vi "Add_Next_Calib_Details.vi"(1 "% Change":dbl format="%.2f", 3 "Hours between calibrations":dbl format="%.2f", 4 "Instrument type":T1=enum."Cross wire velocity", 5 "Calib file Orig":path=path "/Hong(6%)/calib/XW Ch 1 7_10_02_5", 6 "Calib file New":path=path "/Hong(6%)/calib/XW Ch 1 7_10_02_6") -> (0 "Results Files Updated":bool)   [LabVIEW 2010]
uses:
  Controls/Cal_Inst_type.ctl
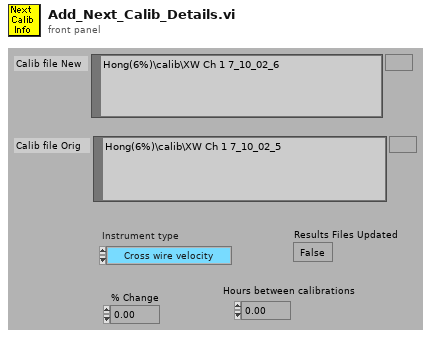
[diagram p1: front panel]
types:
  T1 = typedef "Cal_Inst_type.ctl" = enum16{"Propeller anemometer", "Pressure Transducer", "Hot wire", "Cross wire velocity", "Cross wire angle", "Generic Linear", "Generic Polynomial", "Generic BackPoly", "Fast FID", "Thermocouple", "Cold wire", "Pulsed Wire"}
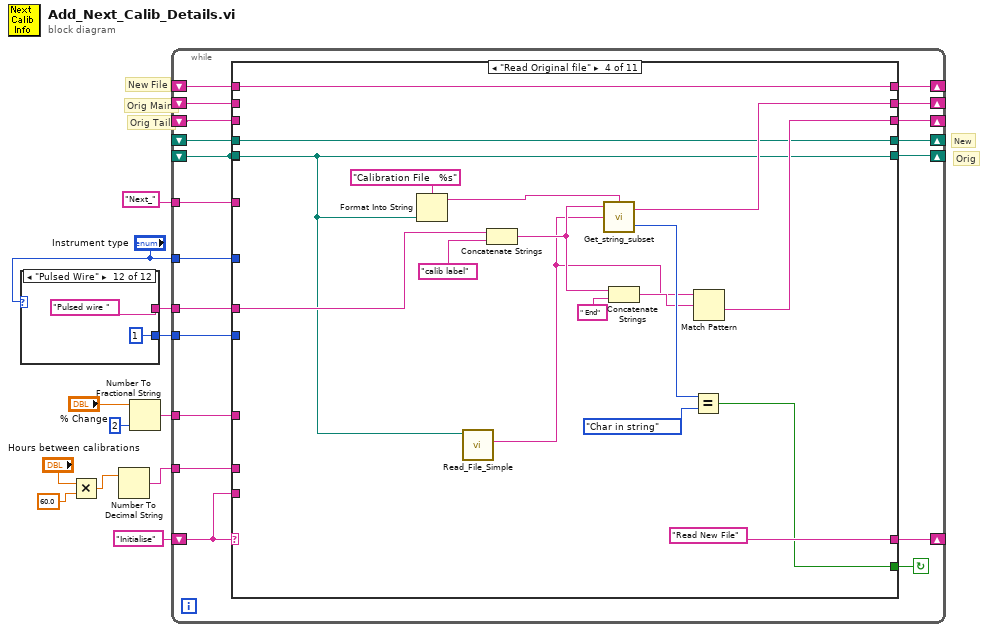
[diagram p0: block diagram]
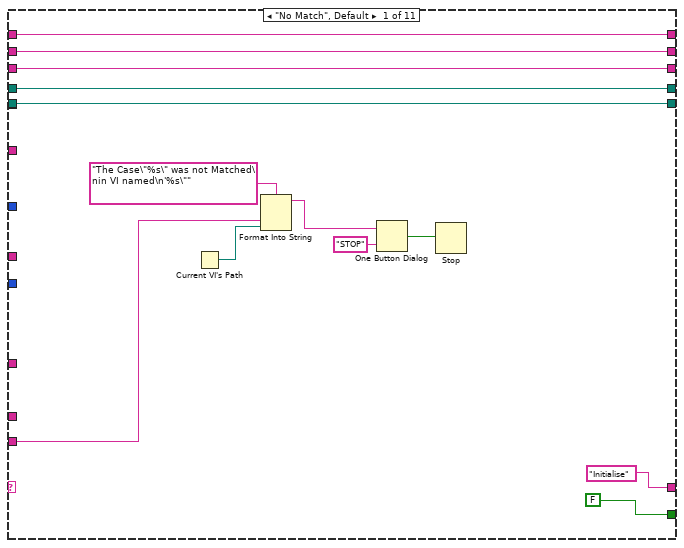
[diagram p2: hidden frame]
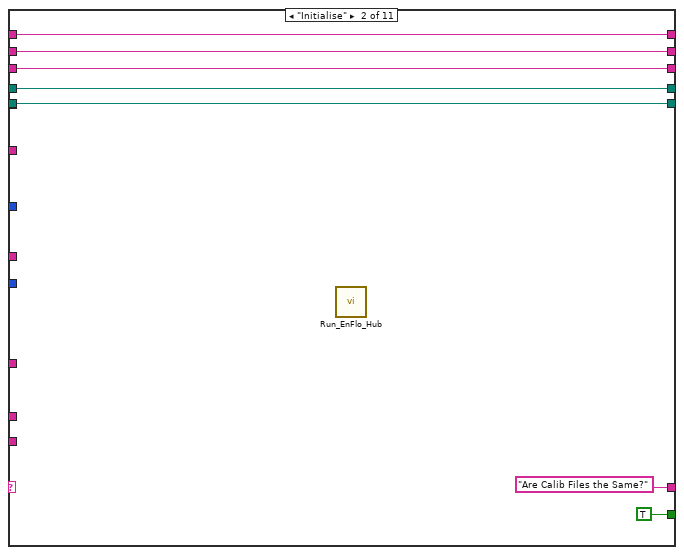
[diagram p3: hidden frame]
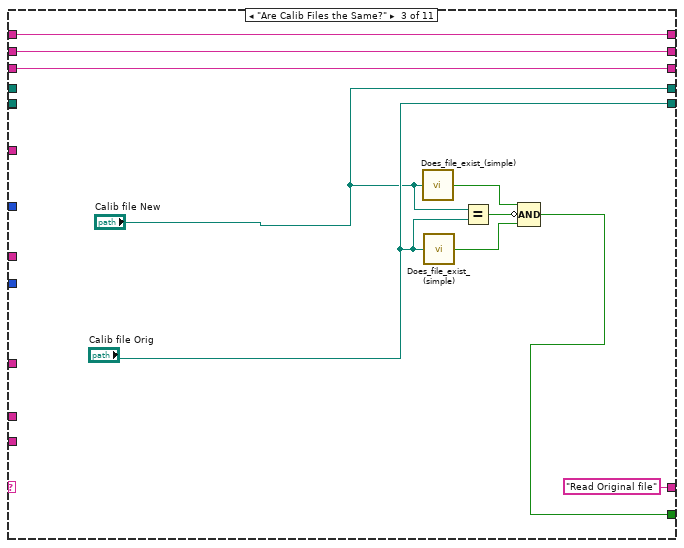
[diagram p4: hidden frame]
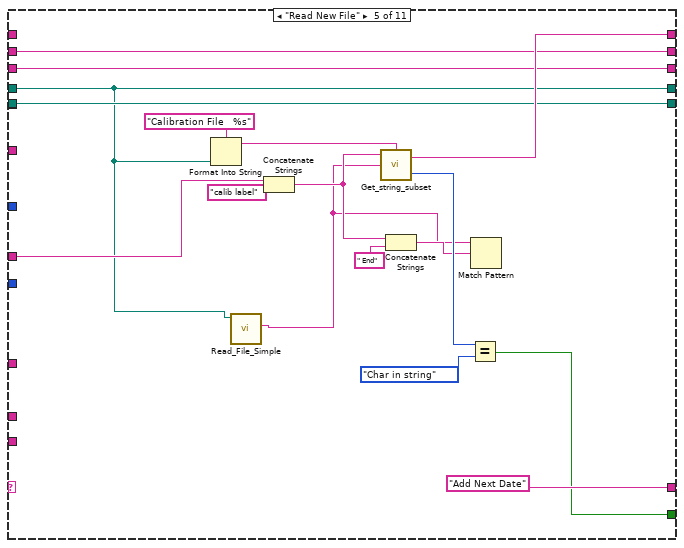
[diagram p5: hidden frame]
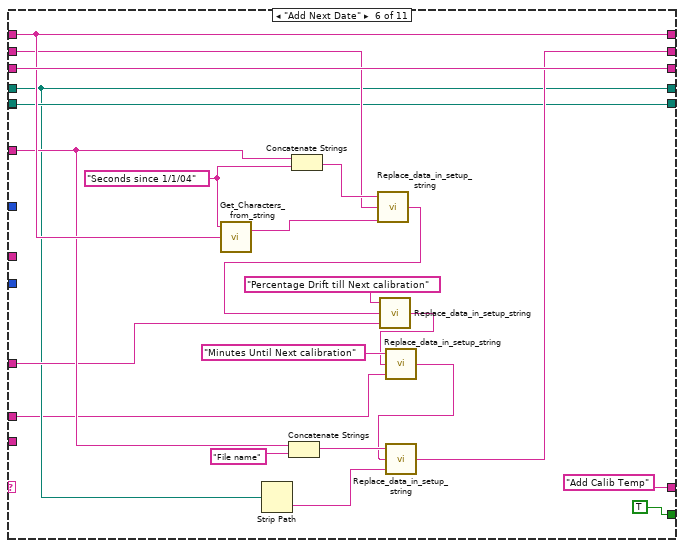
[diagram p6: hidden frame]
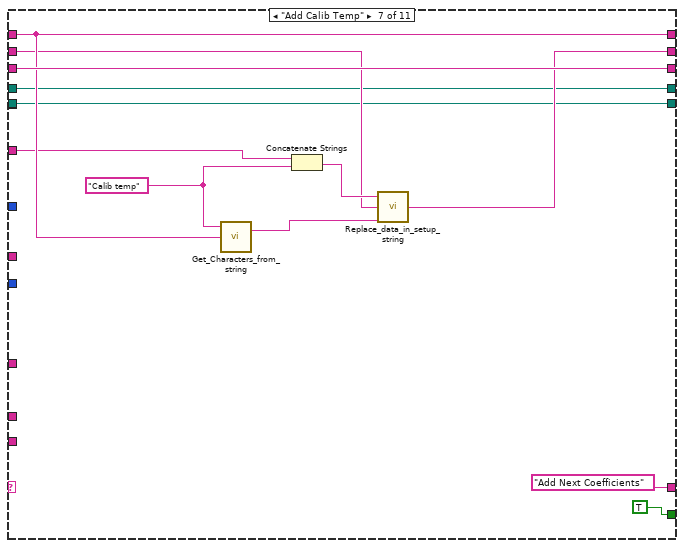
[diagram p7: hidden frame]
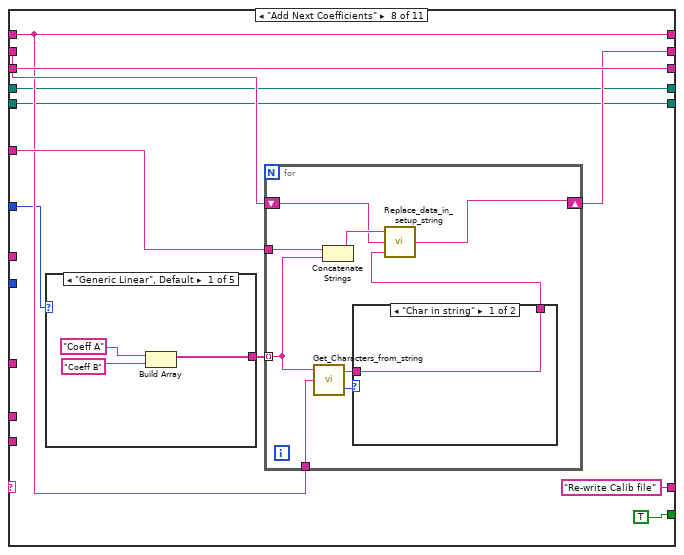
[diagram p8: hidden frame]
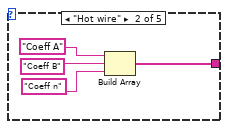
[diagram p9: hidden frame]
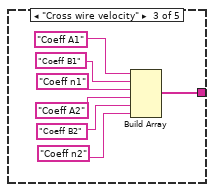
[diagram p10: hidden frame]
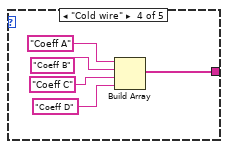
[diagram p11: hidden frame]
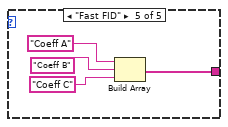
[diagram p12: hidden frame]
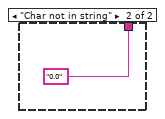
[diagram p13: hidden frame]
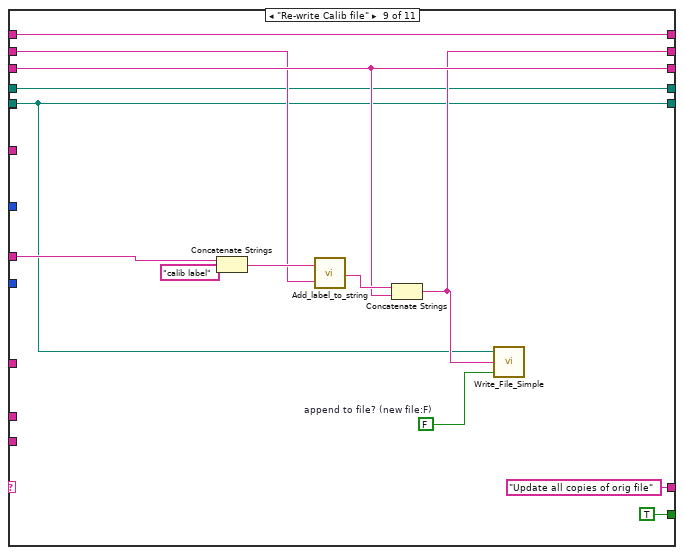
[diagram p14: hidden frame]
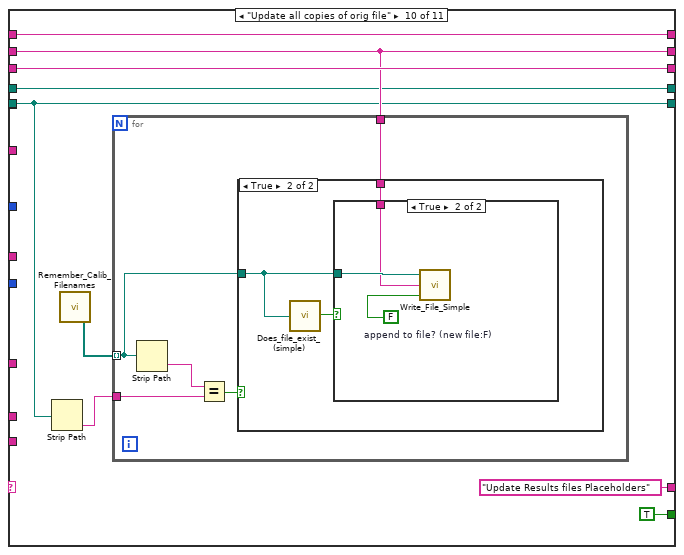
[diagram p15: hidden frame]
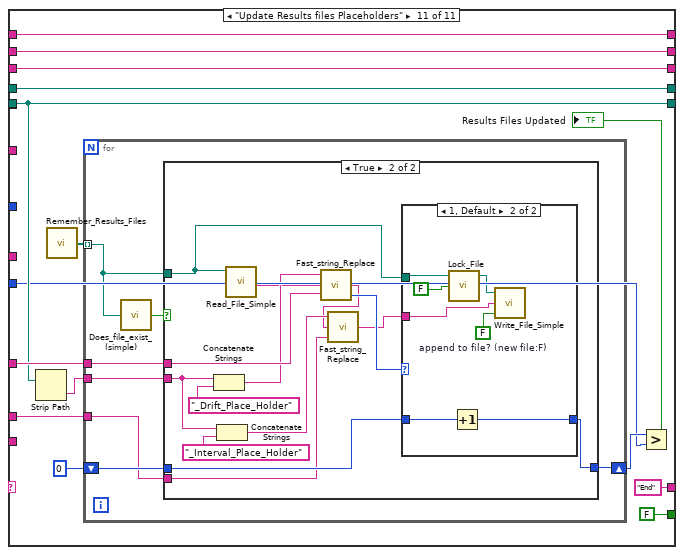
[diagram p18: hidden frame]
diagram:
  # "Orig"
  # "New"
  # "Orig Tail"
  # "New File"
  # "Orig Main"
  n1 = case shown="\"Pulsed Wire\"" "Instrument type" {
    tunnel: ["Prop " "Mano " "HW " "Cross wire velocity " "Cross wire angle " "Generic Inst " "Generic Polynomial " "Generic BackPoly " "Fast FID " "Thermocouple " "Cold wire " "Pulsed wire "] -> w10
    tunnel: [1 ("y") 1 ("y") 1 ("y") 1 ("y") 1 ("y") 1 ("y") 1 ("y") 1 ("y") 3 ("y") 1 ("y") 1 ("y") 1 ("y")] -> w1
    frame "Propeller anemometer" {
    }
    frame "Pressure Transducer" {
    }
    frame "Hot wire" {
    }
    frame "Cross wire velocity" {
    }
    frame "Cross wire angle" {
    }
    frame "Generic Linear" {
    }
    frame "Generic Polynomial" {
    }
    frame "Generic BackPoly" {
    }
    frame "Fast FID" {
    }
    frame "Thermocouple" {
    }
    frame "Cold wire" {
    }
    frame "Pulsed Wire" {
    }
  }
  n2 = Multiply(x="Hours between calibrations", y=60.0) -> (x*y=w3:dbl)
  n3 = Number To Decimal String(number=w3) -> (decimal integer string=w5:string)  [unwired: 1 out]
  n4 = Number To Fractional String(number="% Change", precision (6)=i16 2) -> (F-format string=w6:string)  [unwired: 2 out]
  n5 = while {
    shift-left: _ -> [w39]
    shift-right: [w41] -> _
    shift-left: _ -> [w42]
    shift-right: [w40] -> _
    tunnel: w6 -> [w43]
    tunnel: "Next_" -> [w44]
    tunnel: w10 -> [w45]
    shift-left: _ -> [w46]
    shift-right: [w47] -> _
    shift-left: _ -> [w48]
    shift-right: [w50] -> _
    tunnel: "Instrument type" -> [w52]
    shift-left: _ -> [w49]
    shift-right: [w51] -> _
    shift-left: "Initialise" -> [w53]
    shift-right: [w54] -> _
    tunnel: w5 -> [w38]
    tunnel: w1 -> [w37]
    stop <- w55 continue-if-true
    n6 = case shown="\"Read Original file\"" w53 {
      tunnel: [FALSE TRUE w78 w91 w108 TRUE TRUE TRUE TRUE TRUE FALSE] -> w55
      tunnel: ["Initialise" "Are Calib Files the Same?" "Read Original file" "Read New File" "Add Next Date" "Add Calib Temp" "Add Next Coefficients" "Re-write Calib file" "Update all copies of orig file" "Update Results files Placeholders" "End"] -> w54
      tunnel: w53 -> [w63 _ _ _ _ _ _ _ _ _ _]
      tunnel: w52 -> [_ _ _ _ _ _ _ w157 _ _ _]
      tunnel: [w60 w75 w85 w95 w117 w135 w147 w158 w209 w218 w244] -> w51
      tunnel: [w59 w73 w83 w93 w110 w136 w148 w164 w204 w217 w243] -> w50
      tunnel: w49 -> [w60 w75 w85 w95 _ w135 w147 w158 w209 w218 w244]
      tunnel: w48 -> [w59 w73 w83 _ w110 w136 w148 w164 w204 w217 w243]
      tunnel: [w58 w74 w84 w94 w111 w131 w144 w159 w201 w214 w241] -> w47
      tunnel: w46 -> [w58 w74 w84 _ w111 w134 w146 w160 w202 w214 w241]
      tunnel: w45 -> [_ _ _ w99 w114 _ _ _ w207 _ _]
      tunnel: w44 -> [_ _ _ _ _ w129 w145 w161 _ _ _]
      tunnel: w43 -> [_ _ _ _ _ w126 _ _ _ _ w239]
      tunnel: [w57 w70 "Calib file New" w90 w104 w124 w143 w155 w200 w213 w238] -> w40
      tunnel: [w56 w69 "Calib file Orig" w86 w107 w125 w142 w154 w199 w212 w237] -> w41
      tunnel: w39 -> [w56 w69 _ w86 w107 w125 w142 w154 w199 w212 _]
      tunnel: w42 -> [w57 w70 _ w90 w104 w124 w143 w155 w200 w213 w238]
      tunnel: w39 -> [_ _ _ _ _ _ _ _ _ _ w237]
      tunnel: w38 -> [_ _ _ _ _ w120 _ _ _ _ w235]
      tunnel: w37 -> [_ _ _ _ _ _ _ _ _ _ w232]
      frame "No Match", Default {
        n7 = Current VI's Path() -> (path=w62:path)
        n8 = Format Into String(format string="The Case\"%s\" was not Matched\nin VI named\n'%s\"" ("Format String"), w63, w62) -> (resulting string=w66:string)  [unwired: 2 in, 1 out]
        n9 = One Button Dialog(message=w66, button name ("OK")="STOP") -> (true=w64:bool)
        n10 = Stop(stop? (T)=w64) -> ()
      }
      frame "Initialise" {
        n11 = call "Run_EnFlo_Hub.vi"() -> ()  [unwired: 8 out]
      }
      frame "Are Calib Files the Same?" {
        n12 = call "Does_file_exist_(simple).vi"("Pathname"="Calib file New") -> ("exists?"=w80:bool)
        n13 = call "Does_file_exist_(simple).vi"("Pathname"="Calib file Orig") -> ("exists?"=w79:bool)
        n14 = Equal?(x="Calib file New", y="Calib file Orig") -> (x = y?=w81:bool)
        n15 = Compound Arithmetic op=AND(w80, invert w81, w79) -> (w78:bool)
      }
      frame "Read Original file" {
        n16 = Format Into String(format string="Calibration File   %s", w86) -> (resulting string=w87:string)  [unwired: 2 in, 1 out]
        n17 = call "Read_File_Simple.vi"("Filename"=w86) -> ("string"=w89:string)  [unwired: 2 in, 7 out]
        n18 = Concatenate Strings(w99, "calib label") -> (w96:string)
        n19 = call "Get_string_subset.vi"("String Name"=w87, "String to split"=w89, "File Label"=w96) -> ("Status"=w100:enum16{"Char in string", "Char not in string"}, "Output string"=w94:string)  [unwired: 1 in]
        n20 = Concatenate Strings(w96, " End") -> (w97:string)
        n21 = Equal?(x=w100, y=enum16{"Char in string", "Char not in string"}."Char in string" ("Status")) -> (x = y?=w91:bool)
        n22 = Match Pattern(string=w89, regular expression=w97) -> (after substring=w93:string)  [unwired: 4 out]
      }
      frame "Read New File" {
        n23 = Format Into String(format string="Calibration File   %s", w104) -> (resulting string=w103:string)  [unwired: 2 in, 1 out]
        n24 = call "Read_File_Simple.vi"("Filename"=w104) -> ("string"=w106:string)  [unwired: 2 in, 7 out]
        n25 = Concatenate Strings(w114, "calib label") -> (w109:string)
        n26 = call "Get_string_subset.vi"("String Name"=w103, "String to split"=w106, "File Label"=w109) -> ("Status"=w116:enum16{"Char in string", "Char not in string"}, "Output string"=w117:string)  [unwired: 1 in]
        n27 = Concatenate Strings(w109, " End") -> (w112:string)
        n28 = Equal?(x=w116, y=enum16{"Char in string", "Char not in string"}."Char in string" ("Status")) -> (x = y?=w108:bool)
        n29 = Match Pattern(string=w106, regular expression=w112) -> ()  [unwired: 5 out]
      }
      frame "Add Next Date" {
        w139 = "Seconds since 1/1/04"
        n30 = call "Get_Characters_from_string.vi"("Input string"=w135, "Variable name"=w139) -> ("Value"=w137:string)  [unwired: 1 in, 1 out]
        n31 = Strip Path(path=w124) -> (name=w127:string)  [unwired: 1 out]
        n32 = Concatenate Strings(w129, "File name" ("Variable name")) -> (w128:string)
        n33 = Concatenate Strings(w129, w139) -> (w138:string)
        n34 = call "Replace_data_in_setup_string.vi"("New data string"=w137, "Input string"=w134, "Variable name"=w138) -> ("Appended string"=w132:string)
        n35 = call "Replace_data_in_setup_string.vi"("New data string"=w126, "Input string"=w132, "Variable name"="Percentage Drift till Next calibration") -> ("Appended string"=w122:string)
        n36 = call "Replace_data_in_setup_string.vi"("New data string"=w120, "Input string"=w122, "Variable name"="Minutes Until Next calibration") -> ("Appended string"=w121:string)
        n37 = call "Replace_data_in_setup_string.vi"("New data string"=w127, "Input string"=w121, "Variable name"=w128) -> ("Appended string"=w131:string)
      }
      frame "Add Calib Temp" {
        w151 = "Calib temp"
        n38 = call "Get_Characters_from_string.vi"("Input string"=w147, "Variable name"=w151) -> ("Value"=w149:string)  [unwired: 1 in, 1 out]
        n39 = Concatenate Strings(w145, w151) -> (w150:string)
        n40 = call "Replace_data_in_setup_string.vi"("New data string"=w149, "Input string"=w146, "Variable name"=w150) -> ("Appended string"=w144:string)
      }
      frame "Add Next Coefficients" {
        n41 = case shown="\"Generic Linear\", Default" w157 {
          tunnel: [w165 w168 w172 w179 w184] -> w156
          frame "Generic Linear", Default {
            n42 = Build Array("Coeff A", "Coeff B") -> (w165:string[])
          }
          frame "Hot wire" {
            n43 = Build Array("Coeff A", "Coeff B", "Coeff n") -> (w168:string[])
          }
          frame "Cross wire velocity" {
            n44 = Build Array("Coeff A1", "Coeff B1", "Coeff n1", "Coeff A2", "Coeff B2", "Coeff n2") -> (w172:string[])
          }
          frame "Cold wire" {
            n45 = Build Array("Coeff A", "Coeff B", "Coeff C", "Coeff D") -> (w179:string[])
          }
          frame "Fast FID" {
            n46 = Build Array("Coeff A", "Coeff B", "Coeff C") -> (w184:string[])
          }
        }
        n47 = for {
          tunnel: w156 -> [w195] mode=indexing
          tunnel: w161 -> [w196]
          shift-right: [w192] -> w159
          shift-left: w160 -> [w193]
          tunnel: w158 -> [w188]
          n48 = call "Get_Characters_from_string.vi"("Input string"=w188, "Variable name"=w195) -> ("Status"=w191:enum16{"Char in string", "Char not in string"}, "Value"=w190:string)  [unwired: 1 in]
          n49 = Concatenate Strings(w196, w195) -> (w194:string)
          n50 = case shown="\"Char in string\"" w191 {
            tunnel: w190 -> [w197 _]
            tunnel: [w197 "0.0"] -> w189
            frame "Char in string" {
            }
            frame "Char not in string" {
            }
          }
          n51 = call "Replace_data_in_setup_string.vi"("New data string"=w189, "Input string"=w193, "Variable name"=w194) -> ("Appended string"=w192:string)
        }
      }
      frame "Re-write Calib file" {
        w203 = FALSE  # append to file? (new file:F)
        n52 = Concatenate Strings(w207, "calib label") -> (w206:string)
        n53 = call "Add_label_to_string.vi"("String to write"=w202, "File Label"=w206) -> ("Output string"=w205:string)
        n54 = Concatenate Strings(w205, w204) -> (w201:string)
        n55 = call "Write_File_Simple.vi"("append to file? (new file:F)"=w203, "character string"=w201, "file path"=w199) -> ()  [unwired: 2 out]
      }
      frame "Update all copies of orig file" {
        n56 = Strip Path(path=w212) -> (name=w215:string)  [unwired: 1 out]
        n57 = call "Remember_Calib_Filenames.vi"() -> ("List of Filenames"=w216:path[])  [unwired: 1 in]
        n58 = for {
          tunnel: w216 -> [w222] mode=indexing
          tunnel: w215 -> [w224]
          tunnel: w214 -> [w221]
          n59 = Strip Path(path=w222) -> (name=w225:string)  [unwired: 1 out]
          n60 = Equal?(x=w225, y=w224) -> (x = y?=w223:bool)
          n61 = case shown="True" w223 {
            tunnel: w222 -> [_ w227]
            tunnel: w221 -> [_ w228]
            frame False {
            }
            frame True {
              n62 = call "Does_file_exist_(simple).vi"("Pathname"=w227) -> ("exists?"=w226:bool)
              n63 = case shown="True" w226 {
                tunnel: w227 -> [_ w230]
                tunnel: w228 -> [_ w229]
                frame False {
                }
                frame True {
                  w231 = FALSE  # append to file? (new file:F)
                  n64 = call "Write_File_Simple.vi"("append to file? (new file:F)"=w231, "character string"=w229, "file path"=w230) -> ()  [unwired: 2 out]
                }
              }
            }
          }
        }
      }
      frame "Update Results files Placeholders" {
        n65 = Strip Path(path=w237) -> (name=w240:string)  [unwired: 1 out]
        n66 = call "Remember_Results_Files.vi"() -> ("List of Filenames"=w242:path[])  [unwired: 1 in]
        n67 = for {
          tunnel: w242 -> [w251] mode=indexing
          tunnel: w240 -> [w253]
          tunnel: w239 -> [w252]
          shift-right: [w247] -> w234
          shift-left: 0 -> [w249]
          tunnel: w235 -> [w248]
          n68 = call "Does_file_exist_(simple).vi"("Pathname"=w251) -> ("exists?"=w250:bool)
          n69 = case shown="True" w250 {
            tunnel: w253 -> [_ w259]
            tunnel: w252 -> [_ w268]
            tunnel: w251 -> [_ w263]
            tunnel: [w254 w262] -> w247
            tunnel: w249 -> [w254 w261]
            tunnel: w248 -> [_ w255]
            frame False {
            }
            frame True {
              n70 = Concatenate Strings(w259, "_Drift_Place_Holder" ("Substring")) -> (w266:string)
              n71 = Concatenate Strings(w259, "_Interval_Place_Holder" ("Substring")) -> (w258:string)
              n72 = call "Read_File_Simple.vi"("Filename"=w263) -> ("string"=w265:string)  [unwired: 2 in, 7 out]
              n73 = call "Fast_string_Replace.vi"("Replace match with:"=w268, "Input String"=w265, "regular expression"=w266) -> ("Number Found"=w264:i32, "Output String"=w257:string)  [unwired: 1 out]
              n74 = call "Fast_string_Replace.vi"("Replace match with:"=w255, "Input String"=w257, "regular expression"=w258) -> ("Output String"=w256:string)  [unwired: 2 out]
              n75 = case shown="1, Default" w264 {
                tunnel: w263 -> [_ w273]
                tunnel: w256 -> [_ w270]
                tunnel: [w269 w274] -> w262
                tunnel: w261 -> [w269 w275]
                frame 0 {
                }
                frame 1, Default {
                  w276 = FALSE  # append to file? (new file:F)
                  n76 = call "Lock_File.vi"("Lock File"=FALSE, "path"=w273) -> ("dup path"=w271:path)  [unwired: 1 in, 2 out]
                  n77 = Increment(x=w275) -> (x+1=w274:i32)
                  n78 = call "Write_File_Simple.vi"("append to file? (new file:F)"=w276, "character string"=w270, "file path"=w271) -> ()  [unwired: 2 out]
                }
              }
            }
          }
        }
        n79 = Greater?(x=w234, y=w232) -> (0:→"Results Files Updated":bool)
      }
    }
  }
